vi "retinotopic_map_display_only_120520_svadded.vi"() -> ()   [LabVIEW 2019]
uses:
  <vilib>/Utility/file.llb/Write Delimited Spreadsheet (DBL).vi
panel:
  out "WaitToStop":bool
  in  "Stop":bool
  out "Output":dbl[][](array[numeric])
  out "Display":bool=TRUE
  out "Trial":u32=1
  out "Stimuli Loaded?":bool
  out "Horizontal":bool
  out "stim_id":dbl[](array[numeric])
  out "Vertical":bool
  out "stim_loaded":dbl
  out "Elapsed Time":dbl
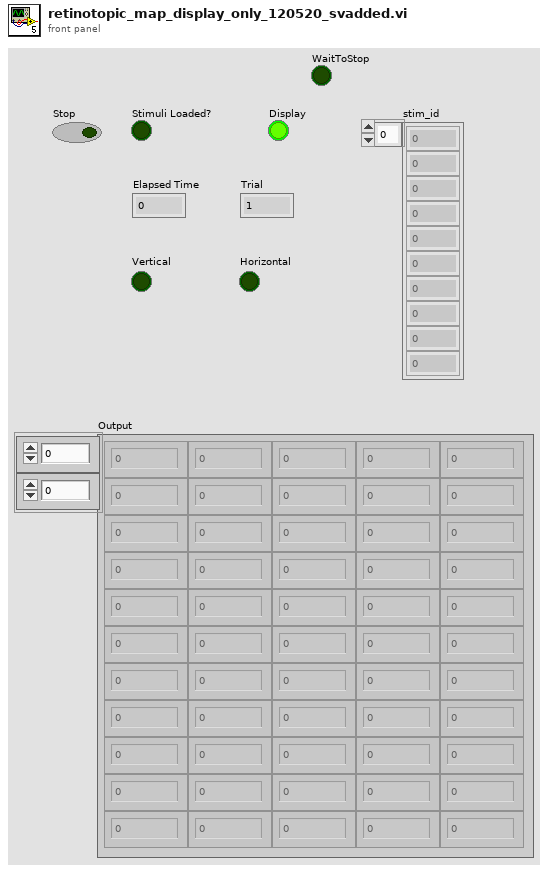
[diagram p1: front panel]
types:
  T1 = typedef "NI_Matrix.lvlib/RealMatrix.ctl" = dbl[][]
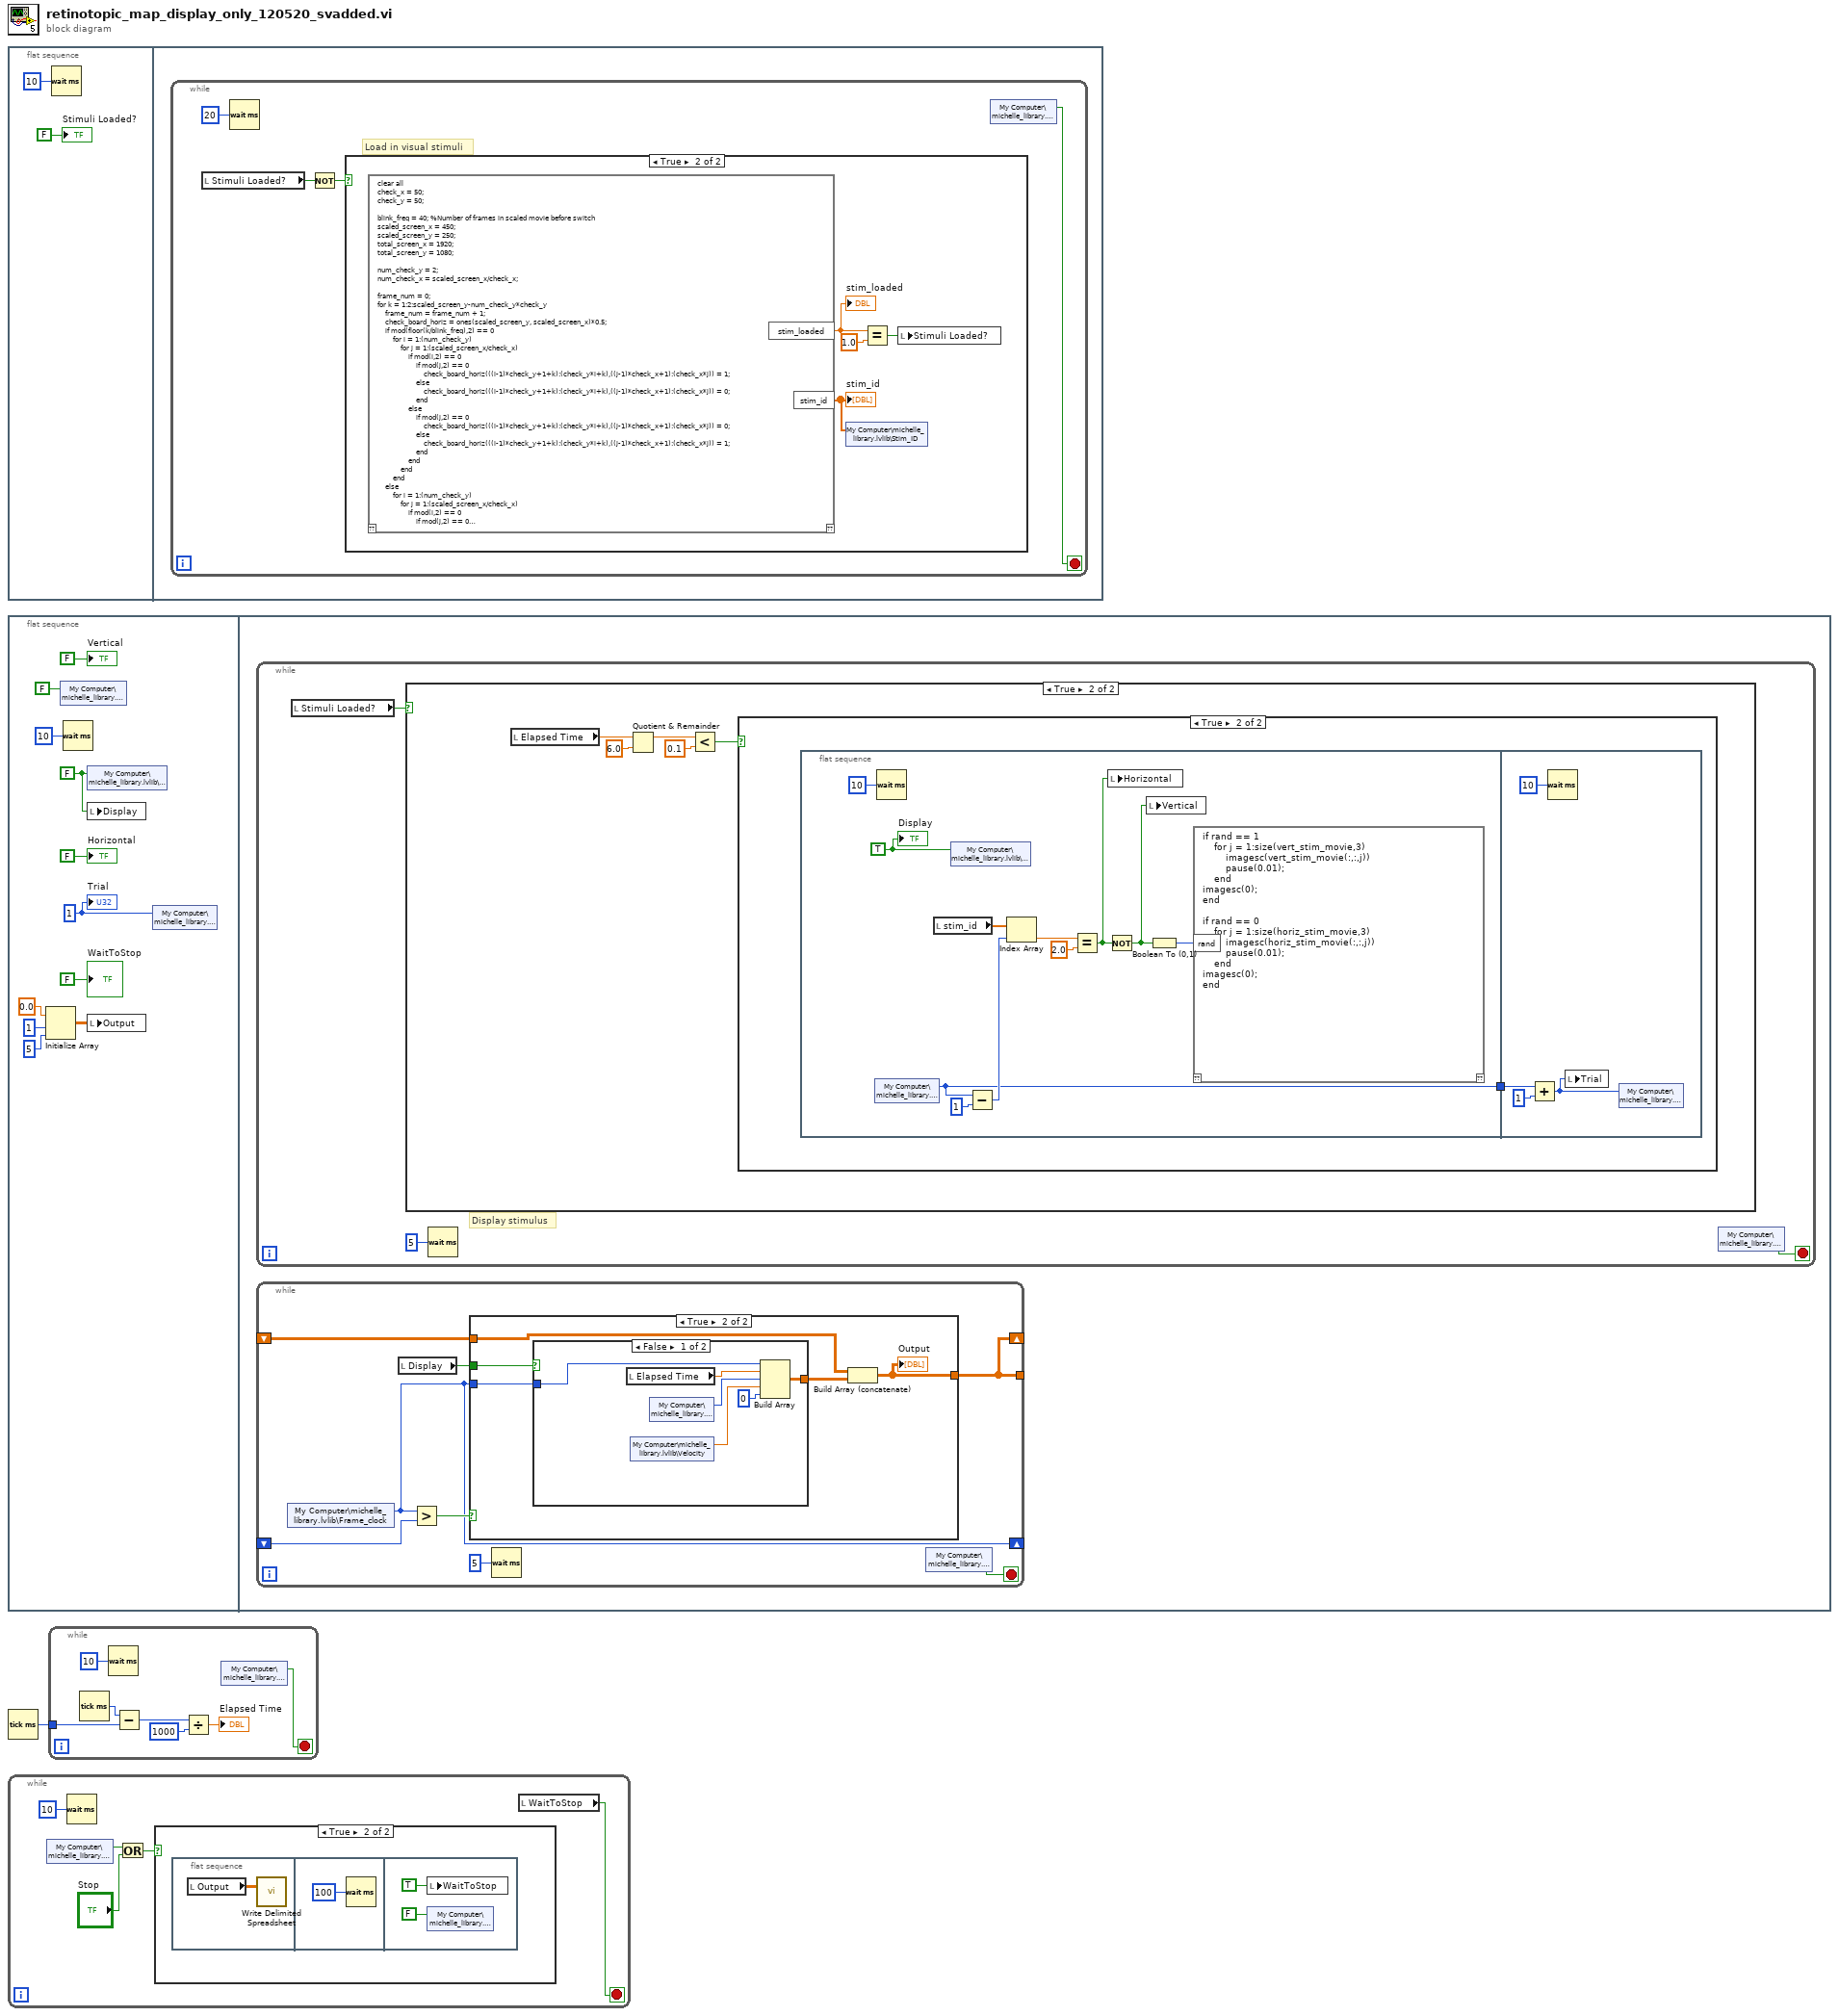
[diagram p0: block diagram]
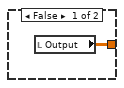
[diagram p4: hidden frame]
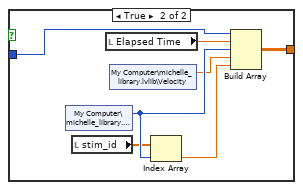
[diagram p5: hidden frame]
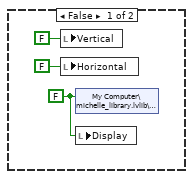
[diagram p7: hidden frame]
diagram:
  n1 = flat-sequence {
    frame #0 {
      n2 = Wait (ms)(milliseconds to wait=u32 10) -> ()  [unwired: 1 out]
      "Stimuli Loaded?" <- FALSE ("Stimuli Loaded?")
    }
    frame #1 {
      n3 = while {
        stop <- w5 stop-if-true
        # "Load in visual stimuli"
        n4 = local read "Stimuli Loaded?"() -> (w4:bool)
        n5 = Wait (ms)(milliseconds to wait=u32 20) -> ()  [unwired: 1 out]
        n6 = Not(x=w4) -> (.not. x?=w7:bool)
        n7 = case shown="True" w7 {
          frame False {
          }
          frame True {
            n8 = script code="clear all\ncheck_x = 50;\ncheck_y = 50;\n\nblink_freq = 40; %Number of frames in scaled movie before switch\nscaled_screen_x = 450;\nscaled_screen_y = 250;\ntotal_screen_x = 1920;\ntotal_screen_y = 1080;\n\nnum_check_y = 2;\nnum_check_x = scaled_screen_x/check_x;\n\nframe_num = 0;\nfor k = 1:2:scaled_screen_y-num_check_y*check_y\n    frame_num = frame_num + 1;\n    check_board_horiz = ones(scaled_screen_y, scaled_screen_x)*0.5;\n    if mod(floor(k/blink_freq),2) == 0\n        for i = 1:(num_check_y)\n            for j = 1:(scaled_screen_x/check_x)\n                if mod(i,2) == 0\n                    if mod(j,2) == 0\n                        check_board_horiz(((i-1)*check_y+1+k):(check_y*i+k),((j-1)*check_x+1):(check_x*j)) = 1;\n                    else\n                        check_board_horiz(((i-1)*check_y+1+k):(check_y*i+k),((j-1)*check_x+1):(check_x*j)) = 0;\n                    end\n                else\n                    if mod(j,2) == 0\n                        check_board_horiz(((i-1)*check_y+1+k):(check_y*i+k),((j-1)*check_x+1):(check_x*j)) = 0;\n                    else\n                        check_board_horiz(((i-1)*check_y+1+k):(check_y*i+k),((j-1)*check_x+1):(check_x*j)) = 1;\n                    end\n                end\n            end\n        end\n    else\n        for i = 1:(num_check_y)\n            for j = 1:(scaled_screen_x/check_x)\n                if mod(i,2) == 0\n                    if mod(j,2) == 0\n                        check_board_horiz(((i-1)*check_y+1+k):(check_y*i+k),((j-1)*check_x+1):(check_x*j)) = 0;\n                    else\n                        check_board_horiz(((i-1)*check_y+1+k):(check_y*i+k),((j-1)*check_x+1):(check_x*j)) = 1;\n                    end\n                else\n                    if mod(j,2) == 0\n                        check_board_horiz(((i-1)*check_y+1+k):(check_y*i+k),((j-1)*check_x+1):(check_x*j)) = 1;\n                    else\n                        check_board_horiz(((i-1)*check_y+1+k):(check_y*i+k),((j-1)*check_x+1):(check_x*j)) = 0;\n                    end\n                end\n            end\n        end\n    end\n    horiz_stim_movie(:,:,frame_num) = check_board_horiz;\nend\n\nnum_check_y = scaled_screen_y/check_y;\nnum_check_x = 2;\n\nframe_num = 0;\nfor k = 1:2:scaled_screen_x-num_check_x*check_x\n    frame_num = frame_num + 1;\n    check_board_vert = ones(scaled_screen_y, scaled_screen_x)*0.5;\n    if mod(floor(k/blink_freq),2) == 0\n        for i = 1:(num_check_x)\n            for j = 1:(scaled_screen_y/check_y)\n                if mod(i,2) == 0\n                    if mod(j,2) == 0\n                        check_board_vert(((j-1)*check_y+1):check_y*j,((i-1)*check_x+1+k):(check_x*i+k)) = 1;\n                    else\n                        check_board_vert(((j-1)*check_y+1):check_y*j,((i-1)*check_x+1+k):(check_x*i+k)) = 0;\n                    end\n                else\n                    if mod(j,2) == 0\n                        check_board_vert(((j-1)*check_y+1):check_y*j,((i-1)*check_x+1+k):(check_x*i+k)) = 0;\n                    else\n                        check_board_vert(((j-1)*check_y+1):check_y*j,((i-1)*check_x+1+k):(check_x*i+k)) = 1;\n                    end\n                end\n            end\n        end\n    else\n        for i = 1:(num_check_x)\n            for j = 1:(scaled_screen_y/check_y)\n                if mod(i,2) == 0\n                    if mod(j,2) == 0\n                        check_board_vert(((j-1)*check_y+1):check_y*j,((i-1)*check_x+1+k):(check_x*i+k)) = 0;\n                    else\n                        check_board_vert(((j-1)*check_y+1):check_y*j,((i-1)*check_x+1+k):(check_x*i+k)) = 1;\n                    end\n                else\n                    if mod(j,2) == 0\n                        check_board_vert(((j-1)*check_y+1):check_y*j,((i-1)*check_x+1+k):(check_x*i+k)) = 1;\n                    else\n                        check_board_vert(((j-1)*check_y+1):check_y*j,((i-1)*check_x+1+k):(check_x*i+k)) = 0;\n                    end\n                end\n            end\n        end\n    end\n    vert_stim_movie(:,:,frame_num) = check_board_vert;\nend\n\nset(0, 'DefaultFigurePosition', [1914 0 1940 2000]);\ncolormap(gray(256))\nset(gcf,'MenuBar','none')\nset(gca,'DataAspectRatioMode','auto')\nset(gca,'Position',[0 0 1 1])\nset(gca, 'xlimmode','manual',...\n           'ylimmode','manual',...\n           'zlimmode','manual',...\n           'climmode','manual',...\n           'alimmode','manual');\nimshow(zeros(total_screen_y,total_screen_x))\n\nstim_id = [ones(1,210)];\naltern = [1:105]*2;\nstim_id(altern) = 2;\nstim_loaded = 1;"() -> ("stim_loaded"=w11:dbl, "stim_id"=w9:dbl[])  [unwired: 1 in, 1 out]
            "stim_loaded" <- w11
            "stim_id" <- w9
            n9 = shared-variable "My Computer\\michelle_library.lvlib\\Stim_ID"(w9) -> ()  [unwired: 1 in, 1 out]
            n10 = Equal?(x=w11, y=1.0) -> (x = y?=w8:bool)
            n11 = local write "Stimuli Loaded?"(w8) -> ()
          }
        }
        n12 = shared-variable "My Computer\\michelle_library.lvlib\\Stop"() -> (w5:bool)  [unwired: 1 in, 1 out]
      }
    }
  }
  n13 = flat-sequence {
    frame #0 {
      w18 = FALSE ("Display")
      w22 = u32 1 ("Trial")
      n14 = Initialize Array(0.0 ("element"), 1 ("dimension size"), 5 ("dimension size")) -> (w14:dbl[][])
      n15 = shared-variable "My Computer\\michelle_library.lvlib\\Stop"(FALSE ("Stop")) -> ()  [unwired: 1 in, 1 out]
      n16 = Wait (ms)(milliseconds to wait=u32 10) -> ()  [unwired: 1 out]
      n17 = shared-variable "My Computer\\michelle_library.lvlib\\Display"(w18) -> ()  [unwired: 1 in, 1 out]
      n18 = local write "Display"(w18) -> ()
      n19 = local write "Output"(w14) -> ()
      n20 = shared-variable "My Computer\\michelle_library.lvlib\\Trial"(w22) -> ()  [unwired: 1 in, 1 out]
      "Horizontal" <- FALSE ("Stimulus 2")
      "Vertical" <- FALSE ("Stimulus 1")
      "Trial" <- w22
      "WaitToStop" <- FALSE
    }
    frame #1 {
      n21 = while {
        stop <- w51 stop-if-true
        # "Display stimulus"
        n22 = local read "Stimuli Loaded?"() -> (w50:bool)
        n23 = case shown="True" w50 {
          frame False {
          }
          frame True {
            n24 = local read "Elapsed Time"() -> (w57:dbl)
            n25 = Quotient & Remainder(x=w57, y=6.0) -> (x-y*floor(x/y)=w55:dbl)  [unwired: 1 out]
            n26 = Less?(x=w55, y=0.1) -> (x < y?=w53:bool)
            n27 = case shown="True" w53 {
              frame False {
                w58 = FALSE ("Display")
                n28 = local write "Vertical"(FALSE) -> ()
                n29 = local write "Horizontal"(FALSE ("Horizontal")) -> ()
                n30 = shared-variable "My Computer\\michelle_library.lvlib\\Display"(w58) -> ()  [unwired: 1 in, 1 out]
                n31 = local write "Display"(w58) -> ()
              }
              frame True {
                n32 = flat-sequence {
                  tunnel: [w63] -> w61
                  tunnel: w61 -> [w76]
                  frame #0 {
                    w67 = TRUE ("Boolean")
                    n33 = shared-variable "My Computer\\michelle_library.lvlib\\Trial"() -> (w63:u32)  [unwired: 1 in, 1 out]
                    n34 = Wait (ms)(milliseconds to wait=u32 10) -> ()  [unwired: 1 out]
                    n35 = local read "stim_id"() -> (w71:dbl[])
                    n36 = shared-variable "My Computer\\michelle_library.lvlib\\Display"(w67) -> ()  [unwired: 1 in, 1 out]
                    n37 = Subtract(x=w63, y=u32 1) -> (x-y=w64:u32)
                    n38 = Index Array(array=w71, index=w64) -> (element=w70:dbl)
                    n39 = Equal?(x=w70, y=2.0) -> (x = y?=w68:bool)
                    n40 = Not(x=w68) -> (.not. x?=w65:bool)
                    n41 = local write "Horizontal"(w68) -> ()
                    n42 = local write "Vertical"(w65) -> ()
                    n43 = Boolean To (0,1)(Boolean=w65) -> (0, 1=w66:i16)
                    n44 = script code="if rand == 1\n    for j = 1:size(vert_stim_movie,3)\n        imagesc(vert_stim_movie(:,:,j))\n        pause(0.01);\n    end\nimagesc(0);\nend\n\nif rand == 0\n    for j = 1:size(horiz_stim_movie,3)\n        imagesc(horiz_stim_movie(:,:,j))\n        pause(0.01);\n    end\nimagesc(0);\nend"("rand"=w66) -> ()  [unwired: 1 in, 1 out]
                    "Display" <- w67
                  }
                  frame #1 {
                    n45 = Add(x=w76, y=u32 1) -> (x+y=w74:u32)
                    n46 = Wait (ms)(milliseconds to wait=u32 10) -> ()  [unwired: 1 out]
                    n47 = local write "Trial"(w74) -> ()
                    n48 = shared-variable "My Computer\\michelle_library.lvlib\\Trial"(w74) -> ()  [unwired: 1 in, 1 out]
                  }
                }
              }
            }
          }
        }
        n49 = Wait (ms)(milliseconds to wait=u32 5) -> ()  [unwired: 1 out]
        n50 = shared-variable "My Computer\\michelle_library.lvlib\\Stop"() -> (w51:bool)  [unwired: 1 in, 1 out]
      }
      n51 = while {
        shift-right: [w25] -> _
        shift-left: _ -> [w30]
        shift-right: [w26] -> _
        shift-left: _ -> [w28]
        tunnel: [w26] -> _
        stop <- w24 stop-if-true
        n52 = shared-variable "My Computer\\michelle_library.lvlib\\Frame_clock"() -> (w25:u32)  [unwired: 1 in, 1 out]
        n53 = local read "Display"() -> (w23:bool)
        n54 = Greater?(x=w25, y=w30) -> (0:w29:bool)
        n55 = case shown="True" w29 {
          tunnel: w25 -> [_ w36]
          tunnel: w28 -> [_ w35]
          tunnel: [w31 w32] -> w26
          tunnel: w23 -> [_ w33]
          frame False {
            n56 = local read "Output"() -> (w31:dbl[][])
          }
          frame True {
            n57 = case shown="False" w33 {
              tunnel: w36 -> [w38 w49]
              tunnel: [w41 w48] -> w34
              frame False {
                n58 = local read "Elapsed Time"() -> (w40:dbl)
                n59 = shared-variable "My Computer\\michelle_library.lvlib\\Velocity"() -> (w37:dbl)  [unwired: 1 in, 1 out]
                n60 = shared-variable "My Computer\\michelle_library.lvlib\\Trial"() -> (w39:u32)  [unwired: 1 in, 1 out]
                n61 = Build Array(w38, w40, w39, w37, 0) -> (w41:T1)
              }
              frame True {
                n62 = shared-variable "My Computer\\michelle_library.lvlib\\Trial"() -> (w46:u32)  [unwired: 1 in, 1 out]
                n63 = local read "stim_id"() -> (w43:dbl[])
                n64 = local read "Elapsed Time"() -> (w47:dbl)
                n65 = shared-variable "My Computer\\michelle_library.lvlib\\Velocity"() -> (w44:dbl)  [unwired: 1 in, 1 out]
                n66 = Index Array(array=w43, index=w46) -> (element=w45:dbl)
                n67 = Build Array(w49, w47, w46, w44, w45) -> (w48:T1)
              }
            }
            n68 = Build Array (concatenate)(w35, w34) -> (w32:T1)
            "Output" <- w32
          }
        }
        n69 = Wait (ms)(milliseconds to wait=u32 5) -> ()  [unwired: 1 out]
        n70 = shared-variable "My Computer\\michelle_library.lvlib\\Stop"() -> (w24:bool)  [unwired: 1 in, 1 out]
      }
    }
  }
  n71 = Tick Count (ms)() -> (millisecond timer value=w1:u32)
  n72 = while {
    stop <- w80 stop-if-true
    n73 = shared-variable "My Computer\\michelle_library.lvlib\\Stop"() -> (w78:bool)  [unwired: 1 in, 1 out]
    n74 = Wait (ms)(milliseconds to wait=u32 10) -> ()  [unwired: 1 out]
    n75 = Or(x=w78, y="Stop") -> (x .or. y?=w77:bool)
    n76 = case shown="True" w77 {
      frame False {
      }
      frame True {
        n77 = flat-sequence {
          frame #0 {
            n78 = local read "Output"() -> (w82:dbl[][])
            n79 = call-poly <vilib>:"Write Delimited Spreadsheet.vi"("2D data"=w82) -> ()  [unwired: 13 in, 2 out]
          }
          frame #1 {
            n80 = Wait (ms)(milliseconds to wait=100) -> ()  [unwired: 1 out]
          }
          frame #2 {
            n81 = local write "WaitToStop"(TRUE) -> ()
            n82 = shared-variable "My Computer\\michelle_library.lvlib\\Stop"(FALSE) -> ()  [unwired: 1 in, 1 out]
          }
        }
      }
    }
    n83 = local read "WaitToStop"() -> (w80:bool)
  }
  n84 = while {
    tunnel: w1 -> [w89]
    stop <- w86 stop-if-true
    n85 = Tick Count (ms)() -> (millisecond timer value=w90:u32)
    n86 = Wait (ms)(milliseconds to wait=u32 10) -> ()  [unwired: 1 out]
    n87 = Subtract(x=w90, y=w89) -> (x-y=w87:u32)
    n88 = Divide(x=w87, y=u32 1000) -> (x/y=→"Elapsed Time":dbl)
    n89 = shared-variable "My Computer\\michelle_library.lvlib\\Stop"() -> (w86:bool)  [unwired: 1 in, 1 out]
  }
